vi "Read ElectrometerConfiguration.vi"(8 "error in (no error)":errorcluster, 11 "Electrometer in":refnum<class "Electrometer.lvclass">) -> (0 "error out":errorcluster, 2 "ElectrometerConfiguration":refnum<class "ElectrometerCOMConfiguration.lvclass">, 3 "Electrometer out":refnum<class "Electrometer.lvclass">)   [LabVIEW 2016, in "Electrometer.lvclass"]
uses:
  Electrometer.lvclass
  ElectrometerConfiguration/ElectrometerCOMConfiguration.lvclass
  Electrometer.lvclass/Electrometer.ctl
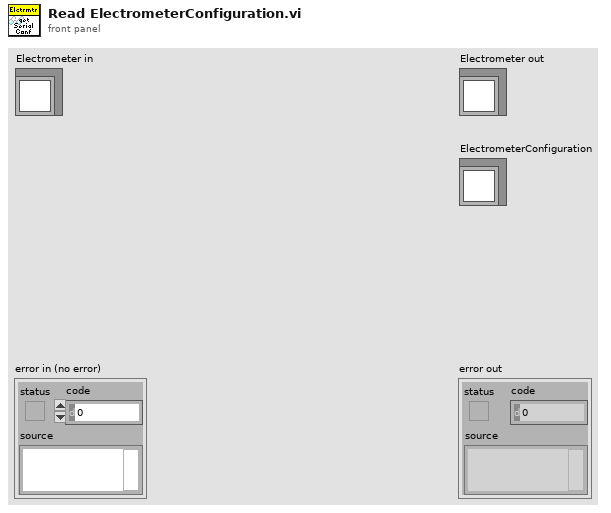
[diagram p1: front panel]
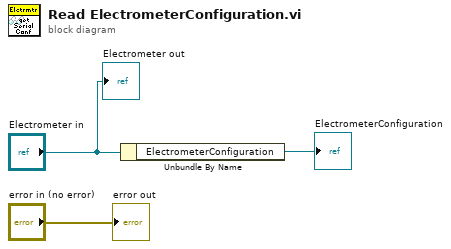
[diagram p0: block diagram]
diagram:
  n1 = Unbundle By Name("Electrometer in") -> ("ElectrometerConfiguration"=→"ElectrometerConfiguration":refnum<class "ElectrometerCOMConfiguration.lvclass">)
  "error out" <- "error in (no error)"
  "Electrometer out" <- "Electrometer in"
